vi "Generate Arduino Data.vi"(8 "error in (no error)":errorcluster, 9 "t0":timestamp, 11 "VISA resource name in":refnum<visa-resource-name>) -> (0 "error out":errorcluster, 1 "next t0":timestamp, 2 "Graph Data":waveform(dbl)[](array[waveform]), 3 "VISA resource name out":refnum<visa-resource-name>)   [LabVIEW 2017, in "Acquisition.lvlib"]
doc: "Generates sample waveforms according to the signal type in the HW Config input."
uses:
  Acquisition.lvlib
panel:
  out "read buffer":string
  out "return count":u32
  out "length":i32
  out "Waveform Chart 2":u32(graph)
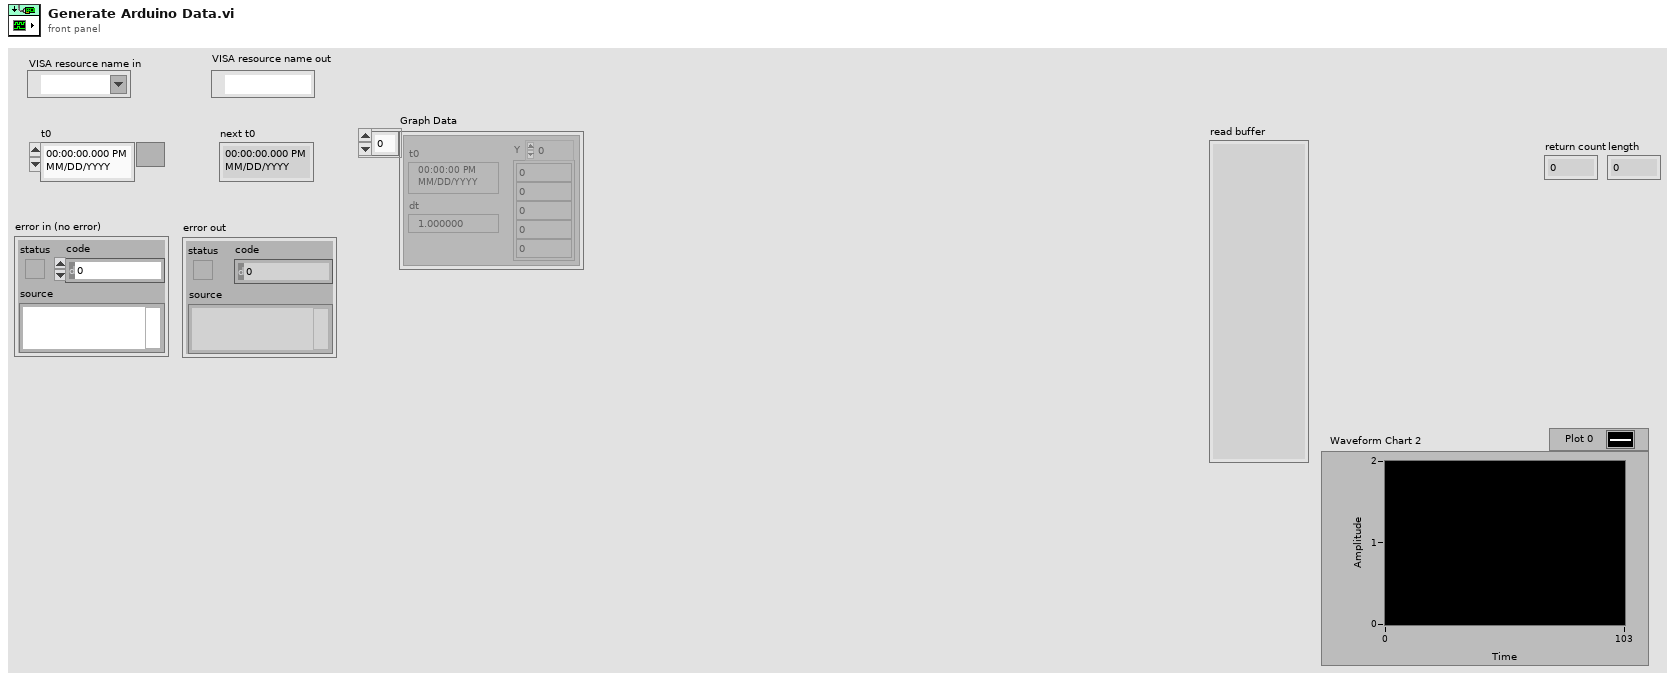
[diagram p1: front panel]
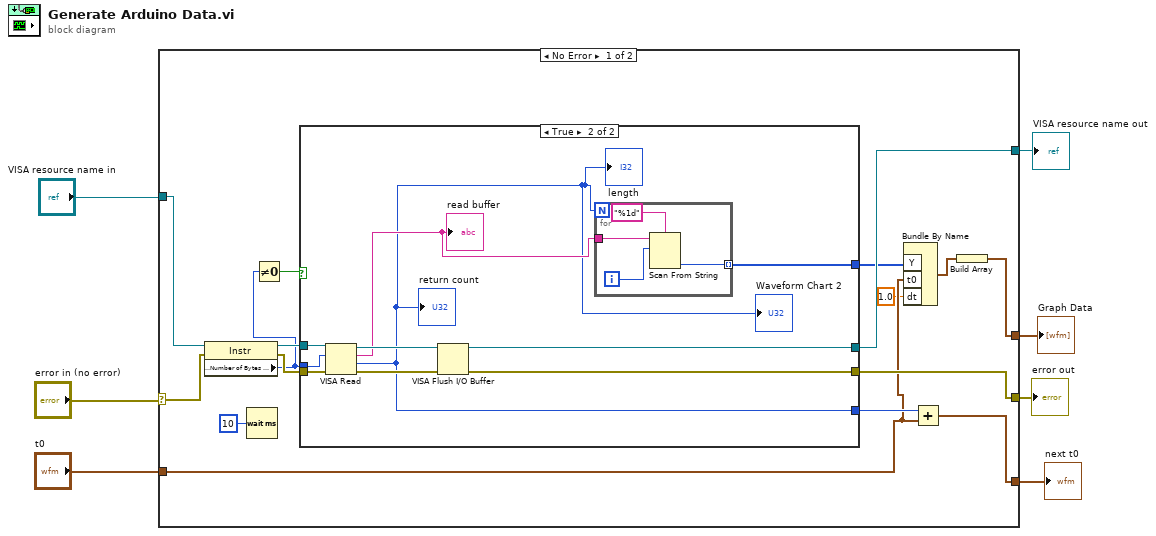
[diagram p0: block diagram]
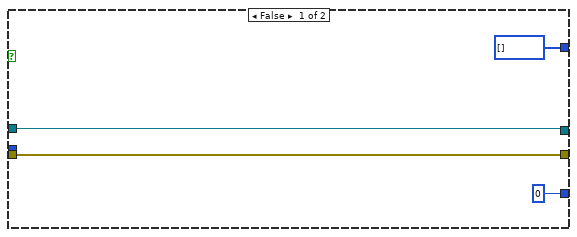
[diagram p2: hidden frame]
diagram:
  n1 = case shown="No Error" "error in (no error)" {
    selector: "error in (no error)" -> [w18 w43]
    tunnel: [w16 w43] -> w6
    tunnel: "VISA resource name in" -> [w19 w42]
    tunnel: [w17 w42] -> w4
    tunnel: [w13 _] -> w3
    tunnel: "t0" -> [w10 _]
    tunnel: [w11 _] -> w1
    frame No Error {
      n2 = property class="Instr"(reference=w19, error in=w18) -> (reference out=w23:refnum<visa-resource-name>, error out=w22:errorcluster, "Serial Settings:Number of Bytes at Serial Port"=w20:u32)
      n3 = Wait (ms)(milliseconds to wait=u32 10) -> ()  [unwired: 1 out]
      n4 = Not Equal To 0?(x=w20) -> (x != 0?=w21:bool)
      n5 = case shown="True" w21 {
        tunnel: w23 -> [w27 w35]
        tunnel: w20 -> [_ w34]
        tunnel: w22 -> [w26 w33]
        tunnel: [w27 w32] -> w17
        tunnel: [w26 w31] -> w16
        tunnel: [i32[] [] w29] -> w15
        tunnel: [u32 0 ("return count") w28] -> w12
        frame False {
        }
        frame True {
          n6 = VISA Read(VISA resource name=w35, byte count=w34, error in (no error)=w33) -> (VISA resource name out=w36:refnum<visa-resource-name>, read buffer=w30:string, return count=w28:u32, error out=w37:errorcluster)
          "read buffer" <- w30
          "return count" <- w28
          "length" <- w28
          "Waveform Chart 2" <- w28
          n7 = VISA Flush I/O Buffer(VISA resource name=w36, error in (no error)=w37) -> (VISA resource name out=w32:refnum<visa-resource-name>, error out=w31:errorcluster)  [unwired: 1 in]
          n8 = for {
            N: w28 -> [_]
            tunnel: w30 -> [w41]
            tunnel: [w38] -> w29 mode=indexing
            i -> [w40]
            n9 = Scan From String(format string="%1d", input string=w41, initial scan location=w40) -> (output 1=w38:i32)  [unwired: 2 in, 3 out]
          }
        }
      }
      n10 = Bundle By Name("Y"=w15, "t0"=w10, "dt"=1.0) -> (w14:waveform(i32))  [unwired: 1 in]
      n11 = Add(x=w12, y=w10) -> (x+y=w11:timestamp)
      n12 = Build Array(w14) -> (w13:waveform(i32)[])
    }
    frame Error {
    }
  }
  "error out" <- w6
  "Graph Data" <- w3
  "VISA resource name out" <- w4
  "next t0" <- w1
